vi "Auswertung_Lichtgitter.vi"(8 "Fehler in":errorcluster, 11 "Cluster in":T1={"Initialisierung"={"Online?"=FALSE, "Grundpfad"=path "", "Kamera Oben"="", "IP-Adresse Flüssiglinse"="", "Flüssiglinse"=refnum, "Kamera Unten"="", "IP-Adresse SPS"="", "SPS-Verbindung"={"TCP Connection Ref"=refnum, "IP address"="", "timeout ms"=5000, "Connected?"=FALSE, "PLC Type"=enum."S7 1200", "Rack S7 400"=0, "Slot S7 400"=0, "PDU Size"=0, "connection semaphore"=refnum}, "IP-Adresse Lichtgitter"="", "Lichtgitter"=refnum, "Skalierungsfaktor"=0.0, "Bilder Oben"=[], "Bild Unten"=refnum, "Bild Ausschnitt Unten"=refnum}, "Einstellungen"={"Gesamtablauf gestartet"=FALSE, "i. O. Bilder speichern"=FALSE, "Bildspeicherung Offline"=FALSE, "Ausgewähltes Offline-Datum"="", "Ausgewähltes Offline-Teil"="", "Speicherpfad Bilder"=path ""}, "Artikeldaten"={"Artikelnummer"="", "Fertigungsauftrag"="", "Muster ISO"=refnum, "Belichtungszeit Referenzmarken"=0.0, "Fokus Referenzmarken"=0.0, "Belichtungszeit ISO"=0.0, "Fokus ISO"=0.0, "Belichtungszeit Unten"=0.0, "Kontaktanzahl"=0, "Aktueller Kontakt"=0, "Kontaktposition"={"x"=0.0, "y"=0.0}, "ISO-Muster nicht vorhanden"=FALSE, "Winkel ISO"=0.0, "Mittelpunkt ISO"={"x"=0.0, "y"=0.0}}, "Werte Kamera Oben"={"Koordinatensystem"={"Punkt x-Achse"={"X"=0.0, "Y"=0.0}, "Ursprung"={"X"=0.0, "Y"=0.0}, "Punkt y-Achse"={"X"=0.0, "Y"=0.0}}, "Position Kontakt"={"x"=0.0, "y"=0.0}, "Durchmesser Loch"=0.0, "Winkel Kontakt"=0.0, "Position Kontakt umgerechnet"={"x"=0.0, "y"=0.0}}, "Werte Kamera Unten"={"Prüfung Unten n. i. O."=FALSE}, "Werte Lichtgitter"={"Messwerte Referenzmarken"=[], "Mittelpunkt Referenzmarken"={"x"=0.0, "y"=0.0}, "Messwerte Kontakt"=[], "Offset"={"x"=0.0, "y"=0.0}}, "Rückmeldungen"={"Koordinaten ermittelt"=FALSE, "Vermessung Lichtgitter fertig"=FALSE, "Nachkontrolle Kamera Unten fertig"=FALSE}, "Fehler"={"Referenzen nicht gefunden"=FALSE, "Kontakt nicht gefunden"=FALSE, "Referenzen nicht in Lichtgitter"=FALSE, "Kontakt zu groß"=FALSE, "Kontakt zu klein"=FALSE}, "Statistik"={"Statistiken"=[]}, "Timer"={"Timer Start Position"=0, "Timer Start Lichtgitter"=0, "Timer Start Kamera Unten"=0}}) -> (0 "Fehler out":errorcluster, 2 "Durchmesser Kontakt (mm)":dbl format="%#.3g", 3 "Cluster out":T1={"Initialisierung"={"Online?"=FALSE, "Grundpfad"=path "", "Kamera Oben"="", "IP-Adresse Flüssiglinse"="", "Flüssiglinse"=refnum, "Kamera Unten"="", "IP-Adresse SPS"="", "SPS-Verbindung"={"TCP Connection Ref"=refnum, "IP address"="", "timeout ms"=5000, "Connected?"=FALSE, "PLC Type"=enum."S7 1200", "Rack S7 400"=0, "Slot S7 400"=0, "PDU Size"=0, "connection semaphore"=refnum}, "IP-Adresse Lichtgitter"="", "Lichtgitter"=refnum, "Skalierungsfaktor"=0.0, "Bilder Oben"=[], "Bild Unten"=refnum, "Bild Ausschnitt Unten"=refnum}, "Einstellungen"={"Gesamtablauf gestartet"=FALSE, "i. O. Bilder speichern"=FALSE, "Bildspeicherung Offline"=FALSE, "Ausgewähltes Offline-Datum"="", "Ausgewähltes Offline-Teil"="", "Speicherpfad Bilder"=path ""}, "Artikeldaten"={"Artikelnummer"="", "Fertigungsauftrag"="", "Muster ISO"=refnum, "Belichtungszeit Referenzmarken"=0.0, "Fokus Referenzmarken"=0.0, "Belichtungszeit ISO"=0.0, "Fokus ISO"=0.0, "Belichtungszeit Unten"=0.0, "Kontaktanzahl"=0, "Aktueller Kontakt"=0, "Kontaktposition"={"x"=0.0, "y"=0.0}, "ISO-Muster nicht vorhanden"=FALSE, "Winkel ISO"=0.0, "Mittelpunkt ISO"={"x"=0.0, "y"=0.0}}, "Werte Kamera Oben"={"Koordinatensystem"={"Punkt x-Achse"={"X"=0.0, "Y"=0.0}, "Ursprung"={"X"=0.0, "Y"=0.0}, "Punkt y-Achse"={"X"=0.0, "Y"=0.0}}, "Position Kontakt"={"x"=0.0, "y"=0.0}, "Durchmesser Loch"=0.0, "Winkel Kontakt"=0.0, "Position Kontakt umgerechnet"={"x"=0.0, "y"=0.0}}, "Werte Kamera Unten"={"Prüfung Unten n. i. O."=FALSE}, "Werte Lichtgitter"={"Messwerte Referenzmarken"=[], "Mittelpunkt Referenzmarken"={"x"=0.0, "y"=0.0}, "Messwerte Kontakt"=[], "Offset"={"x"=0.0, "y"=0.0}}, "Rückmeldungen"={"Koordinaten ermittelt"=FALSE, "Vermessung Lichtgitter fertig"=FALSE, "Nachkontrolle Kamera Unten fertig"=FALSE}, "Fehler"={"Referenzen nicht gefunden"=FALSE, "Kontakt nicht gefunden"=FALSE, "Referenzen nicht in Lichtgitter"=FALSE, "Kontakt zu groß"=FALSE, "Kontakt zu klein"=FALSE}, "Statistik"={"Statistiken"=[]}, "Timer"={"Timer Start Position"=0, "Timer Start Lichtgitter"=0, "Timer Start Kamera Unten"=0}})   [LabVIEW 2024]
doc: "Errechnet aus den Messwerten der Lichtgitter die aktuelle Position des Kontakts, rechnet diese dann in das Koordinatensystem der Kamera um und ermittelt den Offset, welcher von der Achse korrigiert werden muss."
uses:
  Typdefinitionen/Cluster.ctl
  <vilib>/userDefined/High Color/IMAQdx.ctl
  <vilib>/DATA AHEAD/SP7/typedefs/S7 Connection.ctl
  <vilib>/DATA AHEAD/SP7/typedefs/PLC Type.ctl
  <vilib>/vision/Image Controls.llb/IMAQ Image.ctl
  Typdefinitionen/Koordinatensystem.ctl
  Typdefinitionen/Statistik.ctl
  <vilib>/Analysis/Matrix/Datatypes/RealMatrix.ctl
  <vilib>/Analysis/Matrix/Numeric/Conversions/Array To Matrix - RA.vi
  <vilib>/Analysis/Matrix/Numeric/Multiply/Multiply - RM,RM.vi
  <vilib>/Analysis/Matrix/Numeric/Conversions/Matrix To Array - RM.vi
  <vilib>/Utility/file.llb/Write Delimited Spreadsheet (DBL).vi
  <vilib>/Analysis/Matrix/NI_Matrix.lvlib
  <vilib>/DATA AHEAD/SP7/SP7.lvlib
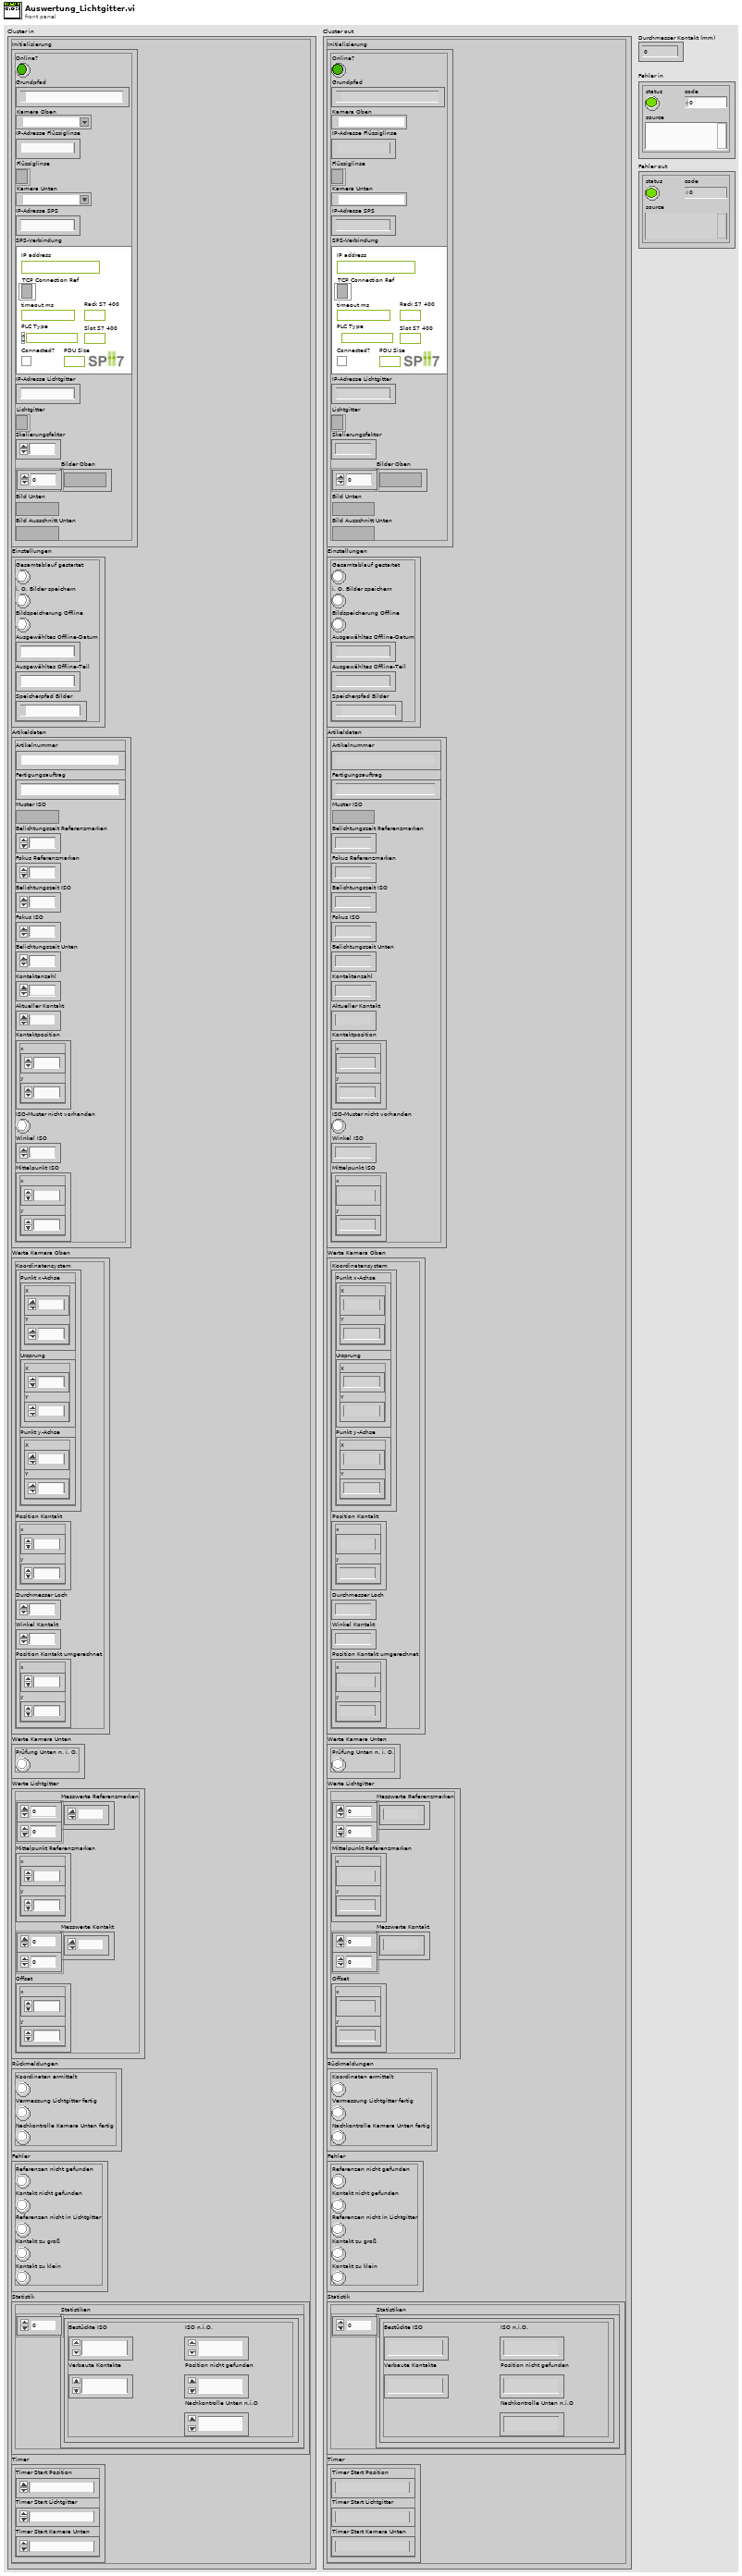
[diagram p1: front panel]
types:
  T1 = typedef "Cluster.ctl" = cluster{"Initialisierung":cluster{"Online?":bool, "Grundpfad":path, "Kamera Oben":T2, "IP-Adresse Flüssiglinse":string, "Flüssiglinse":refnum<k5>, "Kamera Unten":T2, "IP-Adresse SPS":string, "SPS-Verbindung":T3, "IP-Adresse Lichtgitter":string, "Lichtgitter":refnum<k5>, "Skalierungsfaktor":dbl, "Bilder Oben":T6[], "Bild Unten":T6, "Bild Ausschnitt Unten":T6}, "Einstellungen":cluster{"Gesamtablauf gestartet":bool, "i. O. Bilder speichern":bool, "Bildspeicherung Offline":bool, "Ausgewähltes Offline-Datum":string, "Ausgewähltes Offline-Teil":string, "Speicherpfad Bilder":path}, "Artikeldaten":cluster{"Artikelnummer":string, "Fertigungsauftrag":string, "Muster ISO":T6, "Belichtungszeit Referenzmarken":dbl, "Fokus Referenzmarken":dbl, "Belichtungszeit ISO":dbl, "Fokus ISO":dbl, "Belichtungszeit Unten":dbl, "Kontaktanzahl":u32, "Aktueller Kontakt":i16, "Kontaktposition":cluster{"x":sgl, "y":sgl}, "ISO-Muster nicht vorhanden":bool, "Winkel ISO":sgl, "Mittelpunkt ISO":cluster{"x":dbl, "y":dbl}}, "Werte Kamera Oben":cluster{"Koordinatensystem":T7, "Position Kontakt":cluster{"x":dbl, "y":dbl}, "Durchmesser Loch":dbl, "Winkel Kontakt":dbl, "Position Kontakt umgerechnet":cluster{"x":dbl, "y":dbl}}, "Werte Kamera Unten":cluster{"Prüfung Unten n. i. O.":bool}, "Werte Lichtgitter":cluster{"Messwerte Referenzmarken":dbl[][], "Mittelpunkt Referenzmarken":cluster{"x":dbl, "y":dbl}, "Messwerte Kontakt":dbl[][], "Offset":cluster{"x":dbl, "y":dbl}}, "Rückmeldungen":cluster{"Koordinaten ermittelt":bool, "Vermessung Lichtgitter fertig":bool, "Nachkontrolle Kamera Unten fertig":bool}, "Fehler":cluster{"Referenzen nicht gefunden":bool, "Kontakt nicht gefunden":bool, "Referenzen nicht in Lichtgitter":bool, "Kontakt zu groß":bool, "Kontakt zu klein":bool}, "Statistik":cluster{"Statistiken":T8[]}, "Timer":cluster{"Timer Start Position":u32, "Timer Start Lichtgitter":u32, "Timer Start Kamera Unten":u32}}
  T2 = typedef "IMAQdx.ctl" = refnum<k21>
  T3 = typedef "SP7.lvlib/S7 Connection.ctl" = cluster{"TCP Connection Ref":refnum<k5>, "IP address":string, "timeout ms":i32, "Connected?":bool, "PLC Type":T4, "Rack S7 400":u8, "Slot S7 400":u8, "PDU Size":u16, "connection semaphore":T5}
  T4 = typedef "SP7.lvlib/PLC Type.ctl" = enum16{"S7 200", "S7 300/400", "S7 1200", "S7 1500", "LOGO!8"}
  T5 = typedef "Semaphore RefNum" = refnum<k1>
  T6 = typedef "IMAQ Image.ctl" = refnum<image>
  T7 = typedef "Koordinatensystem.ctl" = cluster{"Punkt x-Achse":cluster{"X":sgl, "Y":sgl}, "Ursprung":cluster{"X":sgl, "Y":sgl}, "Punkt y-Achse":cluster{"X":sgl, "Y":sgl}}
  T8 = typedef "Statistik.ctl" = cluster{"Bestückte ISO":u32, "Verbaute Kontakte":u32, "ISO n.i.O.":u32, "Nachkontrolle Unten n.i.O":u32, "Position nicht gefunden":u32}
  T9 = cluster{"Position":cluster{"X":sgl, "Y":sgl}, "Radius":dbl, "Score":dbl}
  T10 = cluster{"Farbe Kreis":u32, "Kreis ausfüllen?":bool, "Bounding Rechteck anzeigen?":bool, "Farbe Bounding Rechteck":u32}
  T11 = typedef "NI_Matrix.lvlib/RealMatrix.ctl" = dbl[][]
  T12 = cluster{"Position":cluster{"X":sgl, "Y":sgl}, "Radius":dbl, "Score":dbl}[]
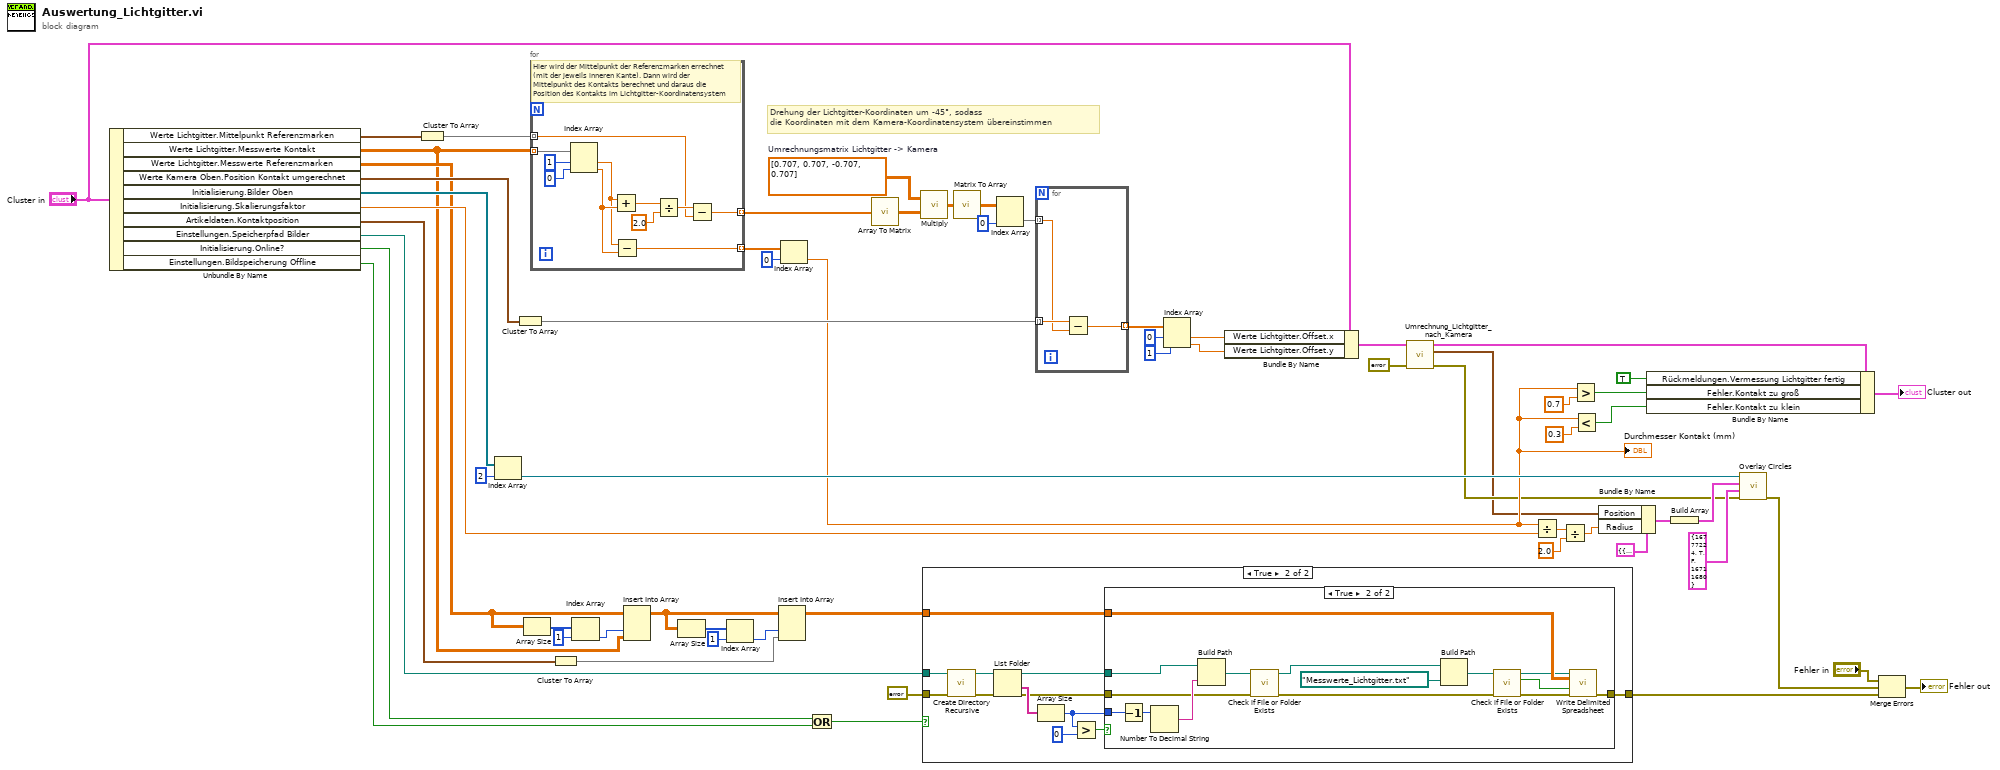
[diagram p0: block diagram]
diagram:
  w62 = T11 [[0.707, 0.707], [-0.707, 0.707]]  # Umrechnungsmatrix Lichtgitter -> Kamera
  # "Drehung der Lichtgitter-Koordinaten um -45°, sodass\ndie Koordinaten mit dem Kamera-Koordinatensystem übereinstimmen"
  n1 = Unbundle By Name("Cluster in") -> ("Werte Lichtgitter.Mittelpunkt Referenzmarken"=w15:cluster{"x":dbl, "y":dbl}, "Werte Lichtgitter.Messwerte Kontakt"=w6:dbl[][], "Werte Lichtgitter.Messwerte Referenzmarken"=w13:dbl[][], "Werte Kamera Oben.Position Kontakt umgerechnet"=w23:cluster{"x":dbl, "y":dbl}, "Initialisierung.Bilder Oben"=w43:T6[], "Initialisierung.Skalierungsfaktor"=w39:dbl, "Artikeldaten.Kontaktposition"=w17:cluster{"x":sgl, "y":sgl}, "Einstellungen.Speicherpfad Bilder"=w46:path, "Initialisierung.Online?"=w19:bool, "Einstellungen.Bildspeicherung Offline"=w16:bool)
  n2 = Cluster To Array(cluster=w15) -> (array=w14:dbl[])
  n3 = Index Array(array=w43, index=2) -> (element=w41:T6)
  n4 = Cluster To Array(cluster=w23) -> (array=w47:dbl[])
  n5 = Array Size(array=w13) -> (size(s)=w22:i32[])
  n6 = for {
    tunnel: w6 -> [w70] mode=indexing
    tunnel: [w74] -> w63 mode=indexing
    tunnel: [w72] -> w50 mode=indexing
    tunnel: w14 -> [w65] mode=indexing
    # "Hier wird der Mittelpunkt der Referenzmarken errechnet (mit der jeweils inneren Kante). Dann wird der Mittelpunkt des Kontakts berechnet und daraus die Position des Kontakts im Lichtgitter-Koordinatensystem"
    n7 = Index Array(array=w70, index #1=1 ("index"), index #2=0 ("index")) -> (element #1=w68:dbl, element #2=w69:dbl)
    n8 = Add(x=w68, y=w69) -> (x+y=w73:dbl)
    n9 = Subtract(x=w68, y=w69) -> (x-y=w72:dbl)
    n10 = Divide(x=w73, y=2.0) -> (x/y=w71:dbl)
    n11 = Subtract(x=w71, y=w65) -> (x-y=w74:dbl)
  }
  n12 = Cluster To Array(cluster=w17) -> (array=w8:sgl[])
  n13 = Index Array(array=w22, index=1) -> (element=w20:i32)
  n14 = Insert Into Array(array=w13, index (col)=w20, new element=w6) -> (w9:dbl[][])  [unwired: 1 in]
  n15 = Array Size(array=w9) -> (size(s)=w10:i32[])
  n16 = Index Array(array=w10, index=1) -> (element=w7:i32)
  n17 = Insert Into Array(array=w9, index (col)=w7, new element=w8) -> (w12:dbl[][])  [unwired: 1 in]
  n18 = Index Array(array=w50, index=0) -> (element=w25:dbl)
  "Durchmesser Kontakt (mm)" <- w25
  n19 = Or(x=w19, y=w16) -> (x .or. y?=w18:bool)
  n20 = call-poly <vilib>:"Array To Matrix.vi"("Real 1D Array"=w63) -> ("Real Matrix (Column Vector)"=w61:T11)
  n21 = call-poly <vilib>:"Multiply.vi"("Real Matrix B"=w61, "Real Matrix A"=w62) -> ("A * B"=w60:T11)
  n22 = case shown="True" w18 {
    tunnel: [w75 w87] -> w52
    tunnel: w46 -> [_ w82]
    tunnel: w12 -> [_ w80]
    tunnel: errorcluster {"status"=FALSE, "code"=0, "source"=""} ("error in") -> [w75 w79]
    frame False {
    }
    frame True {
      n23 = call <vilib>:"Create Directory Recursive.vi"("error in (no error)"=w79, "directory"=w82) -> ("error out"=w85:errorcluster, "directory copy"=w86:path)  [unwired: 3 in, 1 out]
      n24 = List Folder(path=w86, error in=w85) -> (path out=w84:path, folder names=w83:string[], error out=w81:errorcluster)  [unwired: 2 in, 1 out]
      n25 = Array Size(array=w83) -> (size(s)=w78:i32)
      n26 = Greater?(x=w78, y=0) -> (0:w76:bool)
      n27 = case shown="True" w76 {
        tunnel: [w88 w102] -> w87
        tunnel: w84 -> [_ w101]
        tunnel: w78 -> [_ w99]
        tunnel: w81 -> [w88 w97]
        tunnel: w80 -> [_ w94]
        frame False {
        }
        frame True {
          n28 = Decrement(x=w99) -> (x-1=w98:i32)
          n29 = Number To Decimal String(number=w98) -> (decimal integer string=w100:string)  [unwired: 1 in]
          n30 = Build Path(base path=w101, name or relative path=w100) -> (appended path=w96:path)
          n31 = call <vilib>:"Check if File or Folder Exists.vi"("error in (no error)"=w97, "path"=w96) -> ("error out"=w92:errorcluster, "dup path"=w95:path)  [unwired: 7 in, 1 out]
          n32 = Build Path(base path=w95, name or relative path=path "Messwerte_Lichtgitter.txt") -> (appended path=w93:path)
          n33 = call <vilib>:"Check if File or Folder Exists.vi"("error in (no error)"=w92, "path"=w93) -> ("error out"=w89:errorcluster, "file or folder exists?"=w91:bool, "dup path"=w90:path)  [unwired: 7 in]
          n34 = call-poly <vilib>:"Write Delimited Spreadsheet.vi"("file path (dialog if empty)"=w90, "2D data"=w94, "append to file? (new file:F)"=w91, "error in (no error)"=w89) -> ("error out"=w102:errorcluster)  [unwired: 10 in, 1 out]
        }
      }
    }
  }
  n35 = call-poly <vilib>:"Matrix To Array.vi"("Real Matrix"=w60) -> ("Real 2D Array"=w59:dbl[][])
  n36 = Index Array(array=w59, index (col)=0 ("disabled index (col)")) -> (element=w48:dbl[])  [unwired: 1 in]
  n37 = for {
    tunnel: w48 -> [w105] mode=indexing
    tunnel: w47 -> [w106] mode=indexing
    tunnel: [w104] -> w57 mode=indexing
    n38 = Subtract(x=w106, y=w105) -> (x-y=w104:dbl)
  }
  n39 = Index Array(array=w57, index #1=0 ("index"), index #2=1 ("index")) -> (element #1=w44:dbl, element #2=w45:dbl)
  n40 = Bundle By Name(cluster="Cluster in", "Werte Lichtgitter.Offset.x"=w44, "Werte Lichtgitter.Offset.y"=w45) -> (w3:T1)
  n41 = call "Umrechnung_Lichtgitter_nach_Kamera.vi"("error in"=errorcluster {"status"=FALSE, "code"=0, "source"=""}, "Cluster in"=w3) -> ("error out"=w4:errorcluster, "Koordinaten out"=w1:cluster{"X":sgl, "Y":sgl}, "Cluster out"=w2:T1)  [unwired: 7 in]
  n42 = Divide(x=w25, y=w39) -> (x/y=w33:dbl)
  n43 = Divide(x=w33, y=2.0) -> (x/y=w32:dbl)
  n44 = Greater?(x=w25, y=0.7) -> (0:w27:bool)
  n45 = Less?(x=w25, y=0.3) -> (x < y?=w26:bool)
  n46 = Bundle By Name(cluster=T9 {"Position"={"X"=0.0, "Y"=0.0}, "Radius"=0.0, "Score"=0.0} ("Circle Descriptor"), "Position"=w1, "Radius"=w32) -> (w37:T9)
  n47 = Bundle By Name(cluster=w2, "Rückmeldungen.Vermessung Lichtgitter fertig"=TRUE ("Messung Lichtgitter.Vermessung Lichtgitter fertig"), "Fehler.Kontakt zu groß"=w27, "Fehler.Kontakt zu klein"=w26) -> (→"Cluster out":T1)
  n48 = Build Array(w37) -> (w36:T12)
  n49 = call "Overlay Circles.vi"("error in"=w4, "Einstellungen"=T10 {"Farbe Kreis"=16777224, "Kreis ausfüllen?"=TRUE, "Bounding Rechteck anzeigen?"=FALSE, "Farbe Bounding Rechteck"=16711680}, "Circles"=w36, "Image in"=w41) -> ("error out"=w40:errorcluster)  [unwired: 6 in, 1 out]
  n50 = Merge Errors("Fehler in", w40, w52) -> (→"Fehler out":errorcluster)
